vi "hw3.4.vi"() -> ()   [LabVIEW 2014]
panel:
  out "state":string
  in  "Start Button":bool
  in  "stop program":bool
  out "Negative Boolean":bool
  out "ss":dbl
  out "mm":dbl
  out "hh":dbl
  in  "ss":dbl
  in  "mm":dbl
  in  "hh":dbl
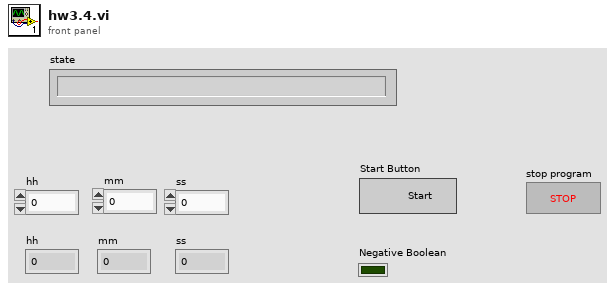
[diagram p1: front panel]
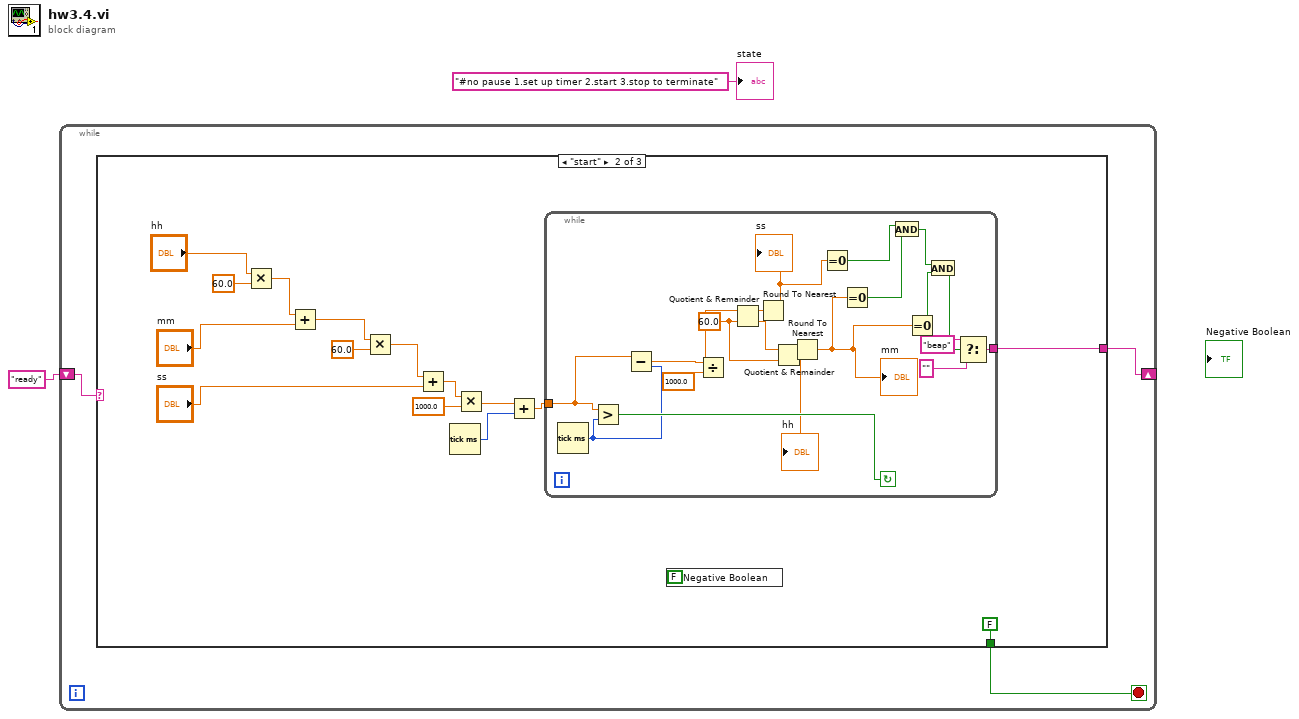
[diagram p0: block diagram]
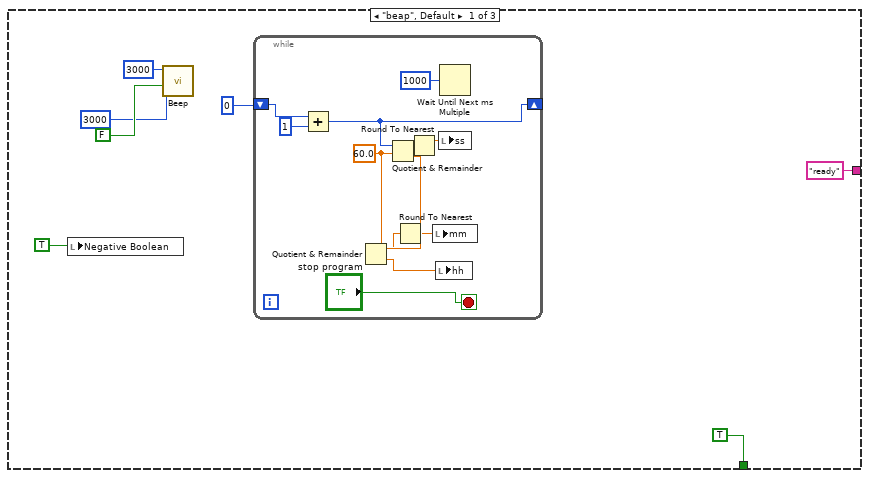
[diagram p2: hidden frame]
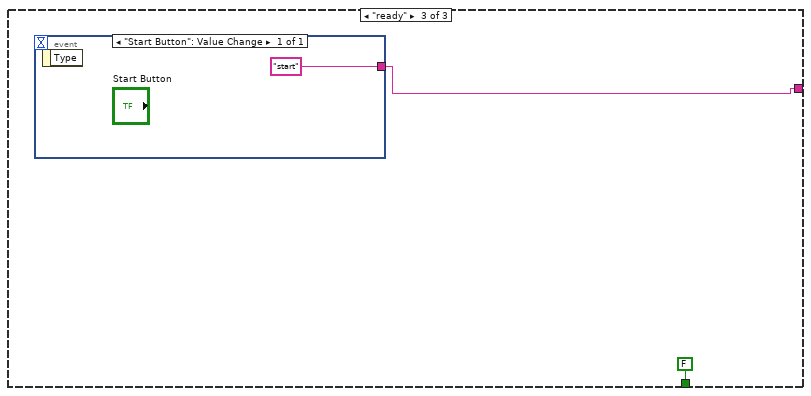
[diagram p3: hidden frame]
diagram:
  n1 = while {
    shift-right: [w4] -> _
    shift-left: "ready" -> [w5]
    stop <- w3 stop-if-true
    n2 = case shown="\"start\"" w5 {
      tunnel: ["ready" w25 w63] -> w4
      tunnel: [TRUE FALSE FALSE] -> w3
      frame "beap", Default {
        n3 = local write "Negative Boolean"(TRUE ("Boolean")) -> ()
        n4 = call <vilib>:"Beep.vi"("use system alert? (T)"=FALSE, "duration (msec)"=u32 3000, "frequency (Hz)"=u32 3000) -> ()  [unwired: 9 in]
        n5 = while {
          shift-right: [w14] -> _
          shift-left: 0 -> [w17]
          stop <- "stop program" stop-if-true
          w21 = 60.0 ("y")
          n6 = Add(x=w17, y=1) -> (x+y=w14:i32)
          n7 = Quotient & Remainder(x=w14, y=w21) -> (x-y*floor(x/y)=w24:dbl, floor(x/y)=w22:dbl)
          n8 = Quotient & Remainder(x=w22, y=w21) -> (x-y*floor(x/y)=w20:dbl, floor(x/y)=w18:dbl)
          n9 = Round To Nearest(number=w20) -> (nearest integer value=w19:dbl)
          n10 = Round To Nearest(number=w24) -> (nearest integer value=w23:dbl)
          n11 = local write "mm"(w19) -> ()
          n12 = local write "hh"(w18) -> ()
          n13 = local write "ss"(w23) -> ()
          n14 = Wait Until Next ms Multiple(millisecond multiple=u32 1000) -> ()  [unwired: 1 out]
        }
      }
      frame "start" {
        n15 = Multiply(x="hh", y=60.0) -> (x*y=w31:dbl)
        n16 = Add(x=w31, y="mm") -> (x+y=w33:dbl)
        n17 = Multiply(x=w33, y=60.0) -> (x*y=w35:dbl)
        n18 = Add(x=w35, y="ss") -> (x+y=w36:dbl)
        n19 = Tick Count (ms)() -> (millisecond timer value=w39:u32)
        n20 = Multiply(x=w36, y=1000.0) -> (x*y=w38:dbl)
        n21 = Add(x=w38, y=w39) -> (x+y=w40:dbl)
        n22 = while {
          tunnel: w40 -> [w41]
          tunnel: [w42] -> w25
          stop <- w61 continue-if-true
          w56 = 60.0 ("y")
          n23 = Tick Count (ms)() -> (millisecond timer value=w60:u32)
          n24 = Greater?(x=w41, y=w60) -> (0:w61:bool)
          n25 = Subtract(x=w41, y=w60) -> (x-y=w59:dbl)
          n26 = Divide(x=w59, y=1000.0) -> (x/y=w53:dbl)
          n27 = Quotient & Remainder(x=w53, y=w56) -> (x-y*floor(x/y)=w58:dbl, floor(x/y)=w57:dbl)
          n28 = Round To Nearest(number=w58) -> (nearest integer value=w51:dbl)
          "ss" <- w51
          n29 = Quotient & Remainder(x=w57, y=w56) -> (x-y*floor(x/y)=w55:dbl, floor(x/y)=→"hh":dbl)
          n30 = Round To Nearest(number=w55) -> (nearest integer value=w47:dbl)
          "mm" <- w47
          n31 = Equal To 0?(x=w51) -> (x = 0?=w50:bool)
          n32 = Equal To 0?(x=w47) -> (x = 0?=w49:bool)
          n33 = And(x=w50, y=w49) -> (x .and. y?=w48:bool)
          n34 = Equal To 0?(x=w47) -> (x = 0?=w46:bool)
          n35 = And(x=w48, y=w46) -> (x .and. y?=w45:bool)
          n36 = Select(t="beap", s=w45, f="") -> (s? t:f=w42:string)
        }
        n37 = local write "Negative Boolean"(FALSE ("Boolean")) -> ()
      }
      frame "ready" {
        n38 = event shown="[0] \"Start Button\": Value Change" {
          selector: _ -> [_]
          dyn-events: _ -> [_]
          timeout: _ -> [_]
          tunnel: ["start"] -> w63
          event "Start Button": Value Change {
            n39 = event-data() -> ()  [unwired: 1 in, 1 out]
          }
        }
      }
    }
  }
  "state" <- "#no pause 1.set up timer 2.start 3.stop to terminate" ("state")
